vi "host.vi"() -> ()   [LabVIEW 2020]
uses:
  <vilib>/Analysis/Matrix/Datatypes/RealMatrix.ctl
  <vilib>/Analysis/baseanly.llb/Mean (DBL).vi
  <vilib>/Analysis/Matrix/Numeric/Conversions/Array To Matrix - RA2.vi
  <vilib>/Analysis/baseanly.llb/Real Inverse Matrix.vi
  <vilib>/Analysis/Matrix/Numeric/Conversions/Matrix To Array - RM.vi
  <vilib>/FPGAPlugInAG/cRIO-9035/niLvFpga_Open_cRIO-9035.vi
  <vilib>/rvi/interface/common/dynamic/niFpgaDynamicAddResources.vi
  <vilib>/Utility/error.llb/Error Cluster From Error Code.vi
  <vilib>/rvi/errors/niLvFpgaAdjustHostInterfaceError.vi
  <vilib>/FPGAPlugInAG/Dynamic/niLvFpga_Run_Dynamic.vi
  <vilib>/FPGAPlugInAG/Dynamic/niLvFpga_Close_Dynamic.vi
  <vilib>/rvi/interface/nirviOpenFPGA/nirviOpenFPGA.xnode
  FPGA Bitfiles/v1.2_FPGATarget_target_16Q3nfesLdw.lvbitx
  target.vi
  <vilib>/rvi/interface/nirviMethod/nirviMethod.xnode
  <vilib>/rvi/interface/nirviReadWriteControl/nirviReadWriteControl.xnode
  <vilib>/rvi/interface/nirviCloseFPGA/nirviCloseFPGA.xnode
  <vilib>/rvi/errors/niLvFpgaMergeErrorWithErrorCode.vi
  <vilib>/Analysis/NI_AALBase.lvlib
  <vilib>/Analysis/Matrix/NI_Matrix.lvlib
  <vilib>/FPGAPlugInAG/Dynamic/niLvFpga_WriteFifo_Dynamic.vi
  <vilib>/FPGAPlugInAG/Dynamic/niLvFpga_ReadFifo_Dynamic.vi
  NiFpgaLv.dll
  <vilib>/rvi/interface/Simulation/niFpgaSimulationCallBeginRW.vi
panel:
  out "percent error":dbl format="%0.2f"
  out "sum of error 2":sgl
  out "divide by zero detected":bool
  out "A":T1
  out "inv(A) LABVIEW-FPGA":sgl[][](array[numeric])
  out "inv(A) LABVIEW":T1
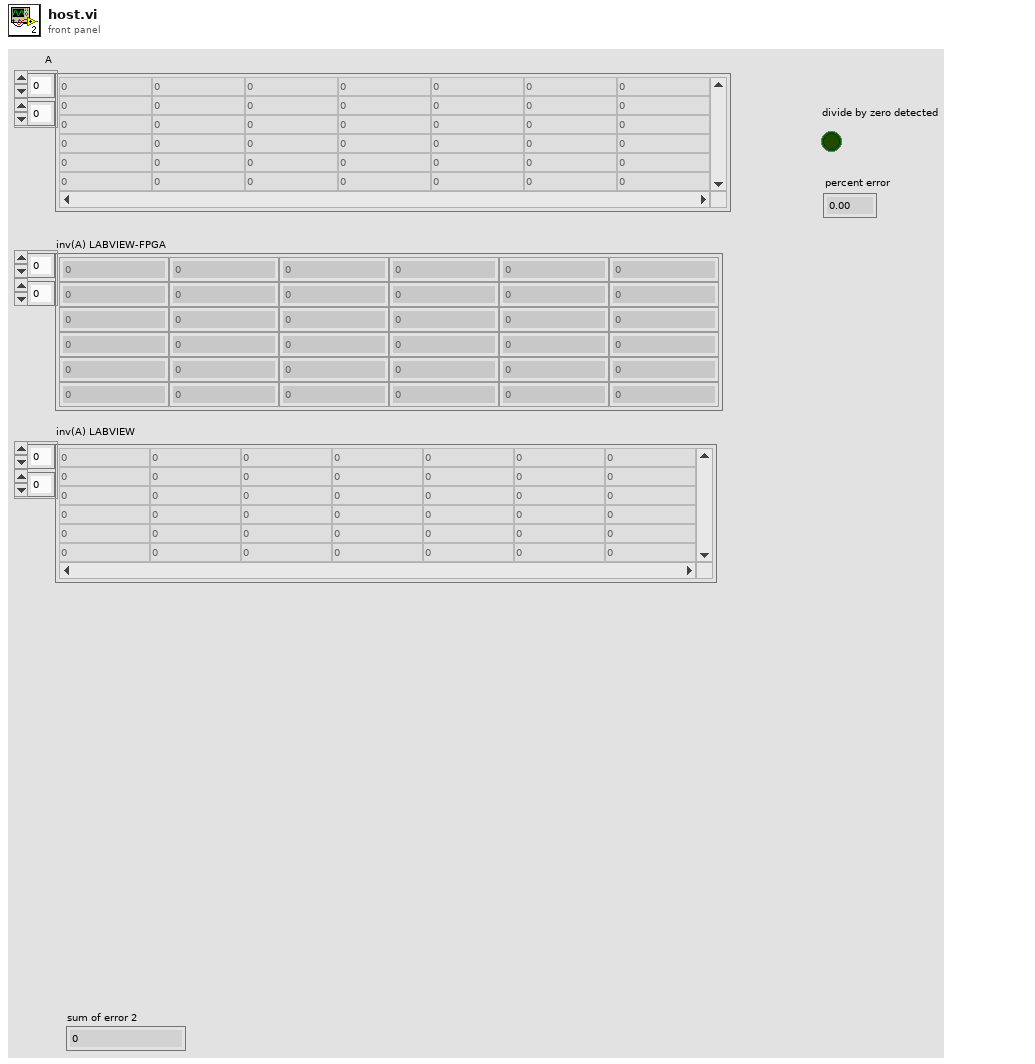
[diagram p1: front panel]
types:
  T1 = typedef "NI_Matrix.lvlib/RealMatrix.ctl" = dbl[][]
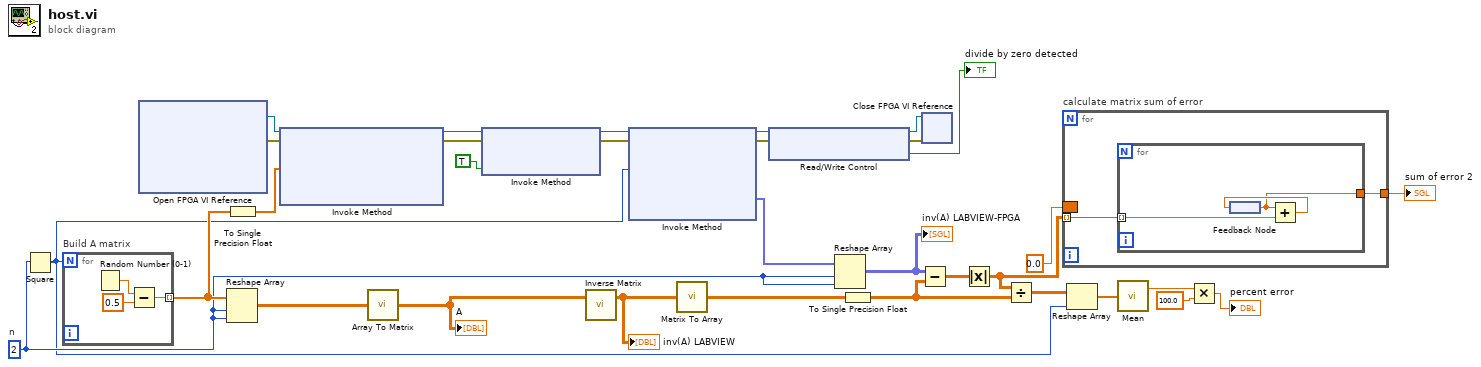
[diagram p0: block diagram]
diagram:
  w5 = 2  # n
  n1 = Square(x=w5) -> (x^2=w2:i32)
  n2 = for "Build A matrix" {
    N: w2 -> [_]
    tunnel: [w33] -> w19 mode=indexing
    n3 = Random Number (0-1)() -> (number: 0 to 1=w35:dbl)
    n4 = Subtract(x=w35, y=0.5) -> (x-y=w33:dbl)
  }
  n5 = xnode "Open FPGA VI Reference"() -> ("FPGA VI Reference Out"=w31:refnum<k20>, "error out"=w30:errorcluster)  [unwired: 2 in]
  n6 = Reshape Array(w19, w5, w5) -> (w21:dbl[][])
  n7 = To Single Precision Float(number=w19) -> (single precision float=w4:sgl[])
  n8 = xnode "Invoke Method"("FPGA VI Reference In"=w31, "error in"=w30, "Data"=w4) -> ("FPGA VI Reference Out"=w27:refnum<k20>, "error out"=w26:errorcluster)  [unwired: 1 in, 1 out]
  n9 = call-poly <vilib>:"Array To Matrix.vi"("Real 2D Array"=w21) -> ("Real Matrix"=w20:T1)
  "A" <- w20
  n10 = xnode "Invoke Method"("FPGA VI Reference In"=w27, "error in"=w26, "Wait Until Done (F)"=TRUE) -> ("FPGA VI Reference Out"=w29:refnum<k20>, "error out"=w28:errorcluster)
  n11 = call-poly <vilib>:"Inverse Matrix.vi"("Input Matrix"=w20) -> ("Inverse Matrix"=w17:T1)  [unwired: 1 in, 1 out]
  "inv(A) LABVIEW" <- w17
  n12 = xnode "Invoke Method"("FPGA VI Reference In"=w29, "error in"=w28, "Number of Elements"=w2) -> ("FPGA VI Reference Out"=w25:refnum<k20>, "error out"=w23:errorcluster, "Data"=w3:fxp<+/-,32,10>[])  [unwired: 1 in, 1 out]
  n13 = call-poly <vilib>:"Matrix To Array.vi"("Real Matrix"=w17) -> ("Real 2D Array"=w16:dbl[][])
  n14 = xnode "Read/Write Control"("FPGA VI Reference In"=w25, "error in"=w23) -> ("FPGA VI Reference Out"=w24:refnum<k20>, "error out"=w22:errorcluster, "divide by zero detected"=→"divide by zero detected":bool)
  n15 = Reshape Array(w3, w5, w5) -> (w14:fxp<+/-,32,10>[][])
  "inv(A) LABVIEW-FPGA" <- w14
  n16 = To Single Precision Float(number=w16) -> (single precision float=w12:sgl[][])
  n17 = Subtract ("Subtract.vi")(x=w14, y=w12) -> (x-y=w18:sgl[][])
  n18 = xnode "Close FPGA VI Reference"("FPGA VI Reference In"=w24, "error in"=w22) -> ()  [unwired: 1 out]
  n19 = Absolute Value ("Absolute Value.vi")(x=w18) -> (abs(x)=w13:sgl[][])
  n20 = Divide(x=w13, y=w12) -> (x/y=w11:sgl[][])
  n21 = for "calculate matrix sum of error" {
    tunnel: w13 -> [w37] mode=indexing
    tunnel: [w36] -> w15
    border: sgl 0.0 -> [_]
    n22 = for {
      tunnel: w37 -> [w40] mode=indexing
      tunnel: [w38] -> w36
      n23 = feedback #1() -> (w38:sgl)
      n24 = Add(x=w38, y=w40) -> (x+y=w39:sgl)
      n25 = feedback-in #1(w39) -> ()
    }
  }
  "sum of error 2" <- w15
  n26 = Reshape Array(w11, w2) -> (w10:sgl[])
  n27 = call-poly <vilib>:"Mean.vi"("X"=w10) -> ("mean"=w9:dbl)  [unwired: 1 out]
  n28 = Multiply(x=w9, y=100.0) -> (x*y=→"percent error":dbl)
